vi "Read Pump Parameters.vi"(8 "error in (no error)":errorcluster, 11 "Pump in":refnum<class "Pump.lvclass">) -> (0 "error out":errorcluster, 2 "Parameters":T1={"Kc"=1.0, "Ti"=0.0, "Td"=0.0, "Min Speed"=0.0, "Max Speed"=100.0}, 3 "Pump out":refnum<class "Pump.lvclass">)   [LabVIEW 2014, in "Pump.lvclass"]
uses:
  Pump.lvclass
  Parameters - cluster.ctl
  <vilib>/JKI/JKI SMO/SMO/SMO.lvclass
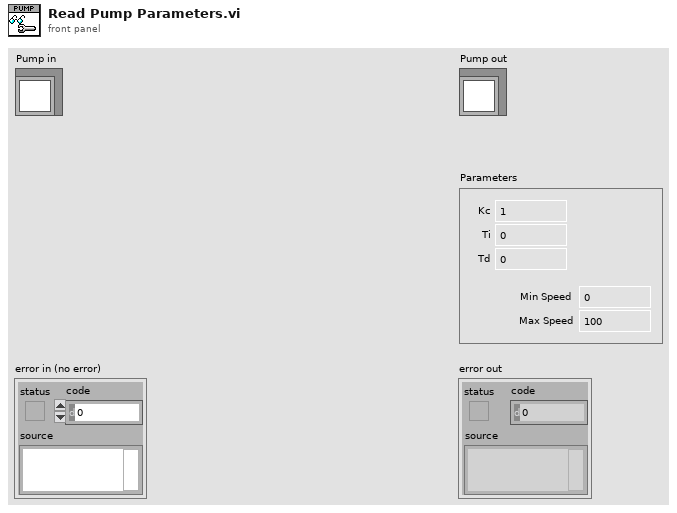
[diagram p1: front panel]
types:
  T1 = typedef "Pump.lvclass/Parameters - cluster.ctl" = cluster{"Kc":dbl, "Ti":dbl, "Td":dbl, "Min Speed":dbl, "Max Speed":dbl}
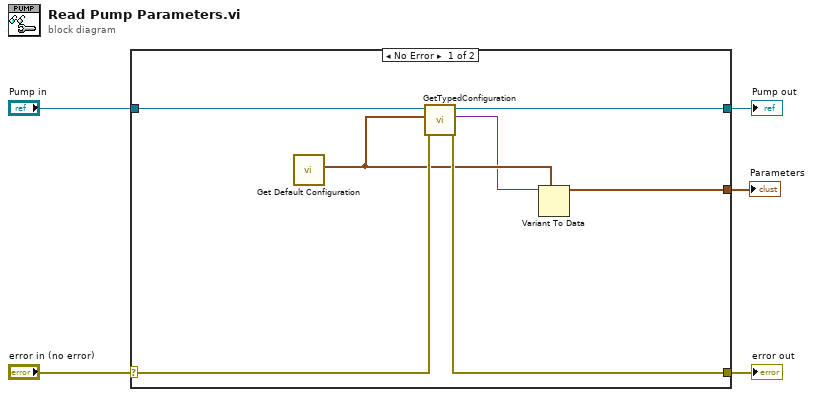
[diagram p0: block diagram]
diagram:
  n1 = case shown="No Error" "error in (no error)" {
    selector: "error in (no error)" -> [w10 w14]
    tunnel: [w9 w14] -> w4
    tunnel: [w11 w13] -> w2
    tunnel: "Pump in" -> [w12 w13]
    tunnel: [w6 _] -> w1
    frame No Error {
      n2 = call "Get Default Configuration.vi"() -> ("Parameters"=w8:T1)  [unwired: 11 in]
      n3 = call <vilib>:"GetTypedConfiguration.vi"("error in (no error)"=w10, "Default value"=w8, "SMO"=w12) -> ("error out"=w9:errorcluster, "Variant"=w7:variant, "SMO out"=w11:refnum<class "Pump.lvclass">)  [unwired: 4 in, 2 out]
      n4 = Variant To Data(type=w8, Variant=w7) -> (data=w6:T1)  [unwired: 1 in, 1 out]
    }
    frame Error {
    }
  }
  "error out" <- w4
  "Pump out" <- w2
  "Parameters" <- w1
